vi "Write Ext by Reference.vi"(8 "Error In":errorcluster, 9 "Data":u8[](array[numeric]), 10 "Type":i8, 11 "Writer In":refnum<data-value>) -> (0 "Error Out":errorcluster, 3 "Writer Out":refnum<data-value>)   [LabVIEW 2018, in "Toolkit.lvlib" / "Writer.lvclass"]
uses:
  Writer.lvclass
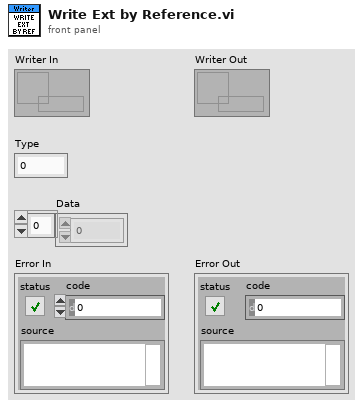
[diagram p1: front panel]
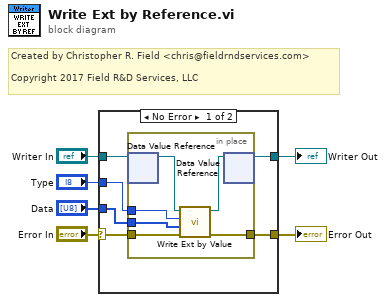
[diagram p0: block diagram]
diagram:
  # "Created by Christopher R. Field <chris@fieldrndservices.com>\n\nCopyright 2017 Field R&D Services, LLC"
  n1 = case shown="No Error" "Error In" {
    selector: "Error In" -> [w10 w20]
    tunnel: [w9 w20] -> w5
    tunnel: "Writer In" -> [w12 w19]
    tunnel: [w11 w19] -> w3
    tunnel: "Data" -> [w8 _]
    tunnel: "Type" -> [w7 _]
    frame No Error {
      n2 = in-place {
        in-place-border: w10 -> [w16]
        in-place-border: [w15] -> w9
        in-place-border: w8 -> [w14]
        in-place-border: w7 -> [w13]
        n3 = in-place-dvr #1(w12) -> (w18:refnum<class "Writer.lvclass">)  [unwired: 1 out]
        n4 = call "Write Ext by Value.vi"("Error In"=w16, "Data"=w14, "Type"=w13, "Writer In"=w18) -> ("Error Out"=w15:errorcluster, "Writer Out"=w17:refnum<class "Writer.lvclass">)  [unwired: 6 in]
        n5 = in-place-dvr #1(w17) -> (w11:refnum<data-value>)  [unwired: 1 out]
      }
    }
    frame Error {
    }
  }
  "Error Out" <- w5
  "Writer Out" <- w3
